vi "IIC Slave Read Bytes.vi"(7 "TimeOutMs":i32, 9 "pReadData":u8[](array[numeric])=array[4097 elements], 10 "IICIndex":i32, 11 "DevHandle":i32) -> (1 "pReadData out":u8[](array[numeric]), 3 "function return":i32)   [LabVIEW 2010, in "usb2iic.lvlib"]
doc: "int WINAPI IIC_SlaveReadBytes(int DevHandle,int IICIndex,unsigned char *pReadData,int TimeOutMs);"
uses:
  usb2iic.lvlib
  USB2XXX.dll
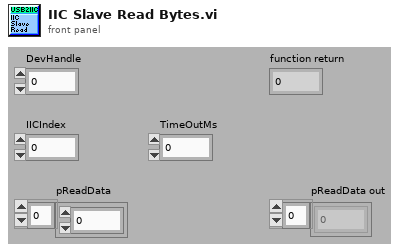
[diagram p1: front panel]
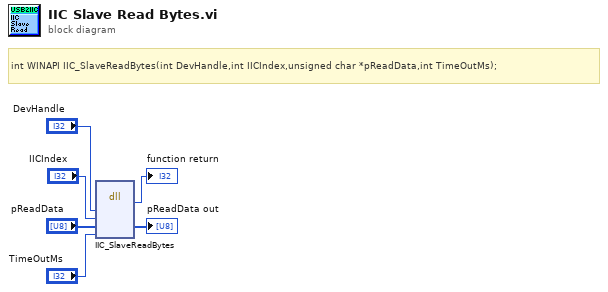
[diagram p0: block diagram]
diagram:
  # "int WINAPI IIC_SlaveReadBytes(int DevHandle,int IICIndex,unsigned char *pReadData,int TimeOutMs);"
  n1 = dll-call lib="G:/OtherWork/USB2XXX_Example/trunk/Labview/PublicFiles/USB2XXX.*" fn="IIC_SlaveReadBytes"("DevHandle"="DevHandle", "IICIndex"="IICIndex", "pReadData"="pReadData", "TimeOutMs"="TimeOutMs") -> (→"function return":i32, "pReadData"=→"pReadData out":u8[])  [unwired: 6 in, 2 out]
